vi "Create_RFID_Baseband_noASK.vi"(5 "Parameters Symbols":T2={"Tari"=2.5e-05, "PW"=0.5, "factor for \"1\" symbol"=0.5, "RTcal"=2.5, "TRcal"=2.5, "Delimiter"=1.25e-05} {"TRcal" min=1.1 max=3.0 step=0.1; "RTcal" min=2.5 max=3.0 step=0.1; "factor for \"1\" symbol" min=0.5 max=1.0 step=0.1; "PW" min=0.265 max=0.525 step=0.001; "Tari" format="%#_3p"}, 7 "Parameters Select":T1={"Target"=0, "Action"=0, "MemBank"=1, "truncate"=FALSE} {"MemBank" items=["00 RFU", "01 EPC", "10 TID", "11 User"]; "Action" items=["000", "001", "010", "011", "100", "101", "110", "111"]; "Target" items=["000 Inventoried (S0)", "001 Inventoried (S1)", "010 Inventoried (S2)", "011 Inventoried (S3)", "100 SL", "101 RFU", "110 RFU", "111 RFU"]}, 9 "Symbol Rate [Hz]":dbl) -> ()   [LabVIEW 2015]
panel:
  out "unsigned 16bit integer":u16[](array[numeric])
  out "Amount of Symbols/Bits":i32
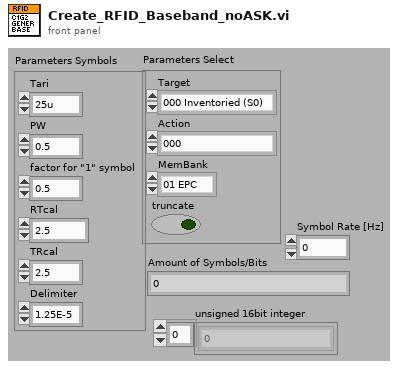
[diagram p1: front panel]
types:
  T1 = cluster{"Target":u16, "Action":u16, "MemBank":u16, "truncate":bool}
  T2 = cluster{"Tari":dbl, "PW":dbl, "factor for \"1\" symbol":dbl, "RTcal":dbl, "TRcal":dbl, "Delimiter":dbl}
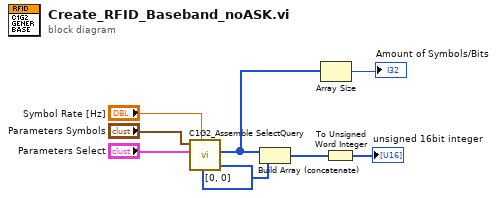
[diagram p0: block diagram]
diagram:
  n1 = call "C1G2_Assemble SelectQuery.vi"("Sample Rate"="Symbol Rate [Hz]", "Parameters Select"="Parameters Select", "Parameters Symbols"="Parameters Symbols") -> ("Signal out"=w3:u8[])  [unwired: 8 in]
  n2 = Build Array (concatenate)(w3, u8[] [0, 0] ("array")) -> (w2:u8[])
  n3 = Array Size(array=w3) -> (size(s)=→"Amount of Symbols/Bits":i32)
  n4 = To Unsigned Word Integer(number=w2) -> (unsigned 16bit integer=→"unsigned 16bit integer":u16[])
